vi "_ConnectorPaneEditor_Get_ vi reference.vi"(8 "error in (no error)":errorcluster, 11 "ConnectorPaneEditor in":refnum<class "_ConnectorPaneEditor.lvclass">) -> (0 "error out":errorcluster, 2 "vi reference":refnum<vi>, 3 "ConnectorPaneEditor out":refnum<class "_ConnectorPaneEditor.lvclass">)   [LabVIEW 2014, in "_ConnectorPaneEditor.lvclass"]
uses:
  _ConnectorPaneEditor.lvclass
  _ConnectorPaneEditor.lvclass/_ConnectorPaneEditor.ctl
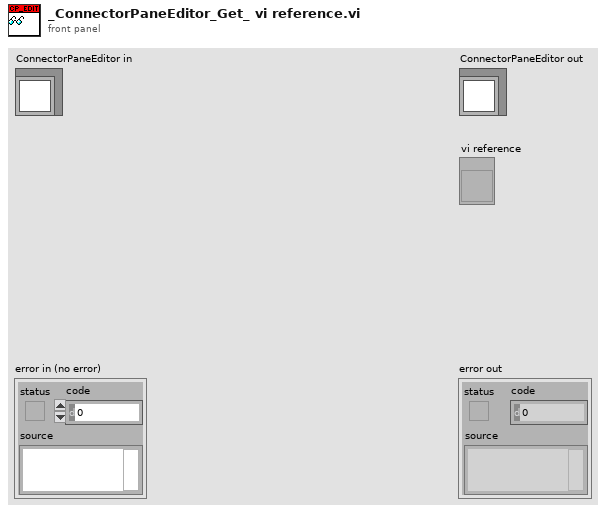
[diagram p1: front panel]
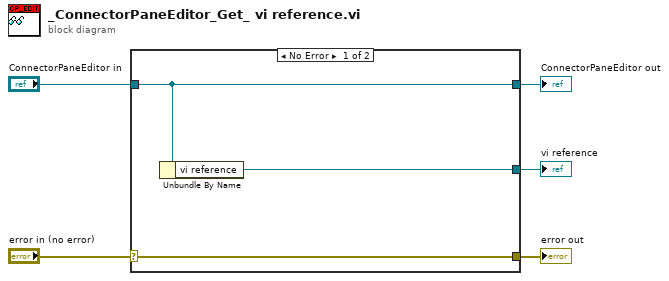
[diagram p0: block diagram]
diagram:
  n1 = case shown="No Error" "error in (no error)" {
    selector: "error in (no error)" -> [w8 w9]
    tunnel: [w8 w9] -> w4
    tunnel: [w7 w10] -> w2
    tunnel: "ConnectorPaneEditor in" -> [w7 w10]
    tunnel: [w6 _] -> w1
    frame No Error {
      n2 = Unbundle By Name(w7) -> ("vi reference"=w6:refnum<vi>)
    }
    frame Error {
    }
  }
  "error out" <- w4
  "ConnectorPaneEditor out" <- w2
  "vi reference" <- w1
